vi "main.vi"() -> ()   [LabVIEW 2023]
uses:
  <vilib>/DAQmx/read.llb/DAQmx Read (Analog 1D DBL NChan 1Samp).vi
  <vilib>/DAQmx/miscellaneous.llb/DAQmx Fill In Error Info.vi
panel:
  out "data":dbl[](array[numeric]) format="%#_6p"
  in  "DAQmx Task Name":refnum<k21>
  out "error out":errorcluster
  in  "error in":errorcluster
  out "Waveform Chart":cluster{"data[0]":dbl, "data[1]":dbl}(graph)
  in  "stop":bool
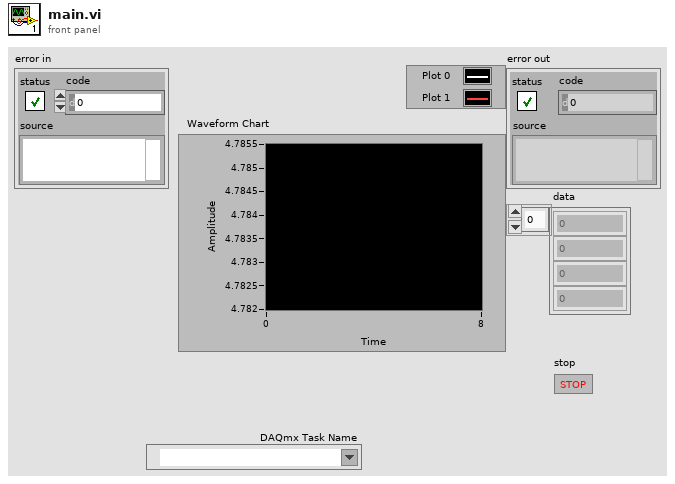
[diagram p1: front panel]
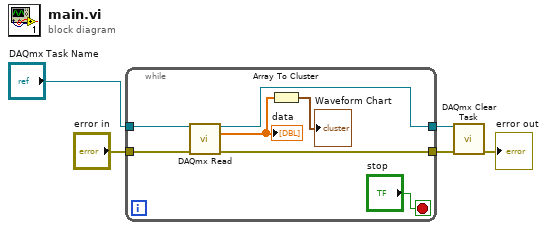
[diagram p0: block diagram]
diagram:
  n1 = while {
    tunnel: "DAQmx Task Name" -> [w11]
    tunnel: "error in" -> [w10]
    tunnel: [w7] -> w3
    tunnel: [w6] -> w2
    stop <- "stop" stop-if-true
    n2 = call-poly <vilib>:"DAQmx Read.vi"("task/channels in"=w11, "error in"=w10) -> ("task out"=w7:refnum<k21>, "data"=w9:dbl[], "error out"=w6:errorcluster)  [unwired: 11 in]
    "data" <- w9
    n3 = Array To Cluster(array=w9) -> (cluster=→"Waveform Chart":cluster{"data[0]":dbl, "data[1]":dbl})
  }
  n4 = call <vilib>:"DAQmx Clear Task.vi"("task in"=w3, "error in"=w2) -> ("error out"=→"error out":errorcluster)  [unwired: 13 in]
